vi "OutputSwerve.vi"() -> ()   [LabVIEW 2023]
doc: "This VI runs feedback and feedforward controllers, manages safety interlocks, and sends commands to the swerve drive and azimuth motors. This VI also controls the commanded drive shifter (low gear or high gear) state."
uses:
  d610c66c-71b6-4d3a-a8b1-b399ee96c8a2.vi
  77f8b8d5-fd7b-4b62-a195-6ccd341d14a1.vi
  e7293d0b-e8ab-4975-ac5b-493dfa430016.vi
  4db519e9-bae7-49f3-a1c3-53a7204bbb79.vi
  6abf8b40-ef0a-49e3-8d46-47362e9bd307.vi
  ae5b7493-7bbf-44c5-8d67-5f44d96a3e48.vi
  744fb9e7-64fc-4bc7-b371-cd49665d8c00.vi
  bd7bff45-d105-4c72-b52f-b7d898b15bf8.vi
  GlobalDriverStationData.vi
  GlobalDrivebase.vi
  GRNF_CTREMotor.vi
  GRNF_GenericSolenoid.vi
  TAI_Motor.vi
  TAI_Solenoid.vi
panel:
  in  "Force To High Gear":bool
  in  "Time Below Speed (ms)":u32=150
  in  "Time Above Speed (ms)":u32=150
  in  "Switch to Low Gear (rpm)":dbl=500.0
  in  "Switch to High Gear (rpm)":dbl=4000.0
  in  "Motor Balancing 3":dbl=0.99
  in  "Motor Balancing 2":dbl=1.0
  in  "Motor Balancing 1":dbl=0.9299999999999999
  in  "Motor Balancing 0":dbl=0.97
  in  "Azimuth PID Parameters":T1={"Kp"=0.2, "Ki"=0.0, "Kd"=10.0, "Kf (don't use)"=0.0, "I-Zone"=10.0} {"Kd" min=0.0; "Ki" min=0.0; "Kp" min=0.0}
  in  "Manual Azimuth Goal (deg) [-180,180]":dbl step=5.0
  in  "Manually Override Azimuth Goal":bool
  in  "Best Angle Hysteresis (deg)":dbl=10.0 format="%#_13g"
  out "Azimuth Position":cluster{dbl, "Interlock Output":dbl}(graph)
  out "Azimuth Error (deg)":dbl
  in  "Plotting":T2(ring)
  in  "Force to Low Gear":bool
  in  "Drive Command Override [0,1]":dbl min=0.0 max=1.0 step=0.1
  in  "Manually Override Drive Command":bool
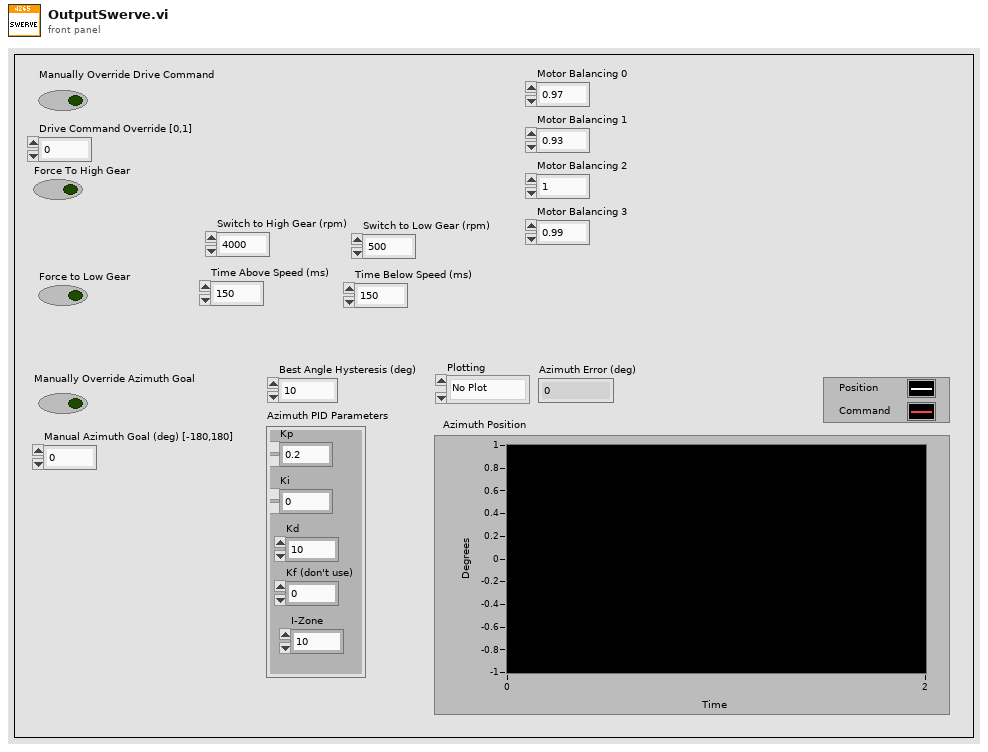
[diagram p1: front panel]
types:
  T1 = cluster{"Kp":dbl, "Ki":dbl, "Kd":dbl, "Kf (don't use)":dbl, "I-Zone":dbl}
  T2 = enum16{"No Plot", "Module 0", "Module 1", "Module 2", "Module 3"}
  T3 = enum16{"Safety", "Travelling", "Positioning", "Holding"}
  T4 = typedef "WPI_MotorControlDeviceRef.ctl" = cluster{"DeviceStatus":errorcluster, "Type":T5, "PWM":cluster{"PWM Channel":T6, "DeadBand":T7}, "CAN":cluster{"Device Number":u8, "SetOutput VI Ref":variant, "GetOutput VI Ref":variant, "Enable VI Ref":variant, "Disable VI Ref":variant, "Data":variant}, "Invert":bool, "DIO PWM":cluster{"PWM \"Enable\" Channel":T6, "DIOChannel":T8, "PWM Rate":dbl}}
  T5 = typedef "WPI_MotorControlType.ctl" = enum16{"PWM", "CAN", "DIO PWM"}
  T6 = typedef "FPGA_DIOPWMChannel.ctl" = enum8{"PWM 0", "PWM 1", "PWM 2", "PWM 3", "PWM 4", "PWM 5", "PWM 6", "PWM 7", "PWM 8", "PWM 9", "PWM MXP 0", "PWM MXP 1", "PWM MXP 2", "PWM MXP 3", "PWM MXP 4", "PWM MXP 5", "PWM MXP 6", "PWM MXP 7", "PWM MXP 8", "PWM MXP 9", "Invalid"}
  T7 = typedef "WPI_PWMDeadband.ctl" = cluster{"Name":string, "maxPositivePwm":i32, "minPositivePwm":i32, "centerPwm":i32, "maxNegativePwm":i32, "minNegativePwm":i32, "angularRange":u16}
  T8 = typedef "FPGA_DIOChannel.ctl" = enum8{"DIO 0", "DIO 1", "DIO 2", "DIO 3", "DIO 4", "DIO 5", "DIO 6", "DIO 7", "DIO 8", "DIO 9", "DIO MXP 0", "DIO MXP 1", "DIO MXP 2", "DIO MXP 3", "DIO MXP 4", "DIO MXP 5", "DIO MXP 6", "DIO MXP 7", "DIO MXP 8", "DIO MXP 9", "DIO MXP 10", "DIO MXP 11", "DIO MXP 12", "DIO MXP 13", "DIO MXP 14", "DIO MXP 15", "SPI Port CS1", "SPI Port CS2", "SPI Port CS3", "SPI Port MISO", "SPI Port MOSI", "Invalid"}
  T9 = enum16{"No Changed Output", "New Normal Output", "New Testing Output"}
  T10 = enum16{"Low Gear", "High Gear", "Transiting", "Unknown", "Force Low Gear"}
  T11 = cluster{"SEN_Azimuth_Position_Unwrapped_3 (deg)":dbl, dbl}
  T12 = typedef "WPI_SolenoidDevRef.ctl" = cluster{"DevStatus":errorcluster, "Pneumatics Control Module":u8, "Forward Solenoid Channel":T13, "Reverse Solenoid Channel":T13}
  T13 = typedef "WPI_SolenoidChannel.ctl" = enum8{"Solenoid 0", "Solenoid 1", "Solenoid 2", "Solenoid 3", "Solenoid 4", "Solenoid 5", "Solenoid 6", "Solenoid 7", "Solenoid 8", "Solenoid 9", "Solenoid 10", "Solenoid 11", "Solenoid 12", "Solenoid 13", "Solenoid 14", "Solenoid 15", "Invalid"}
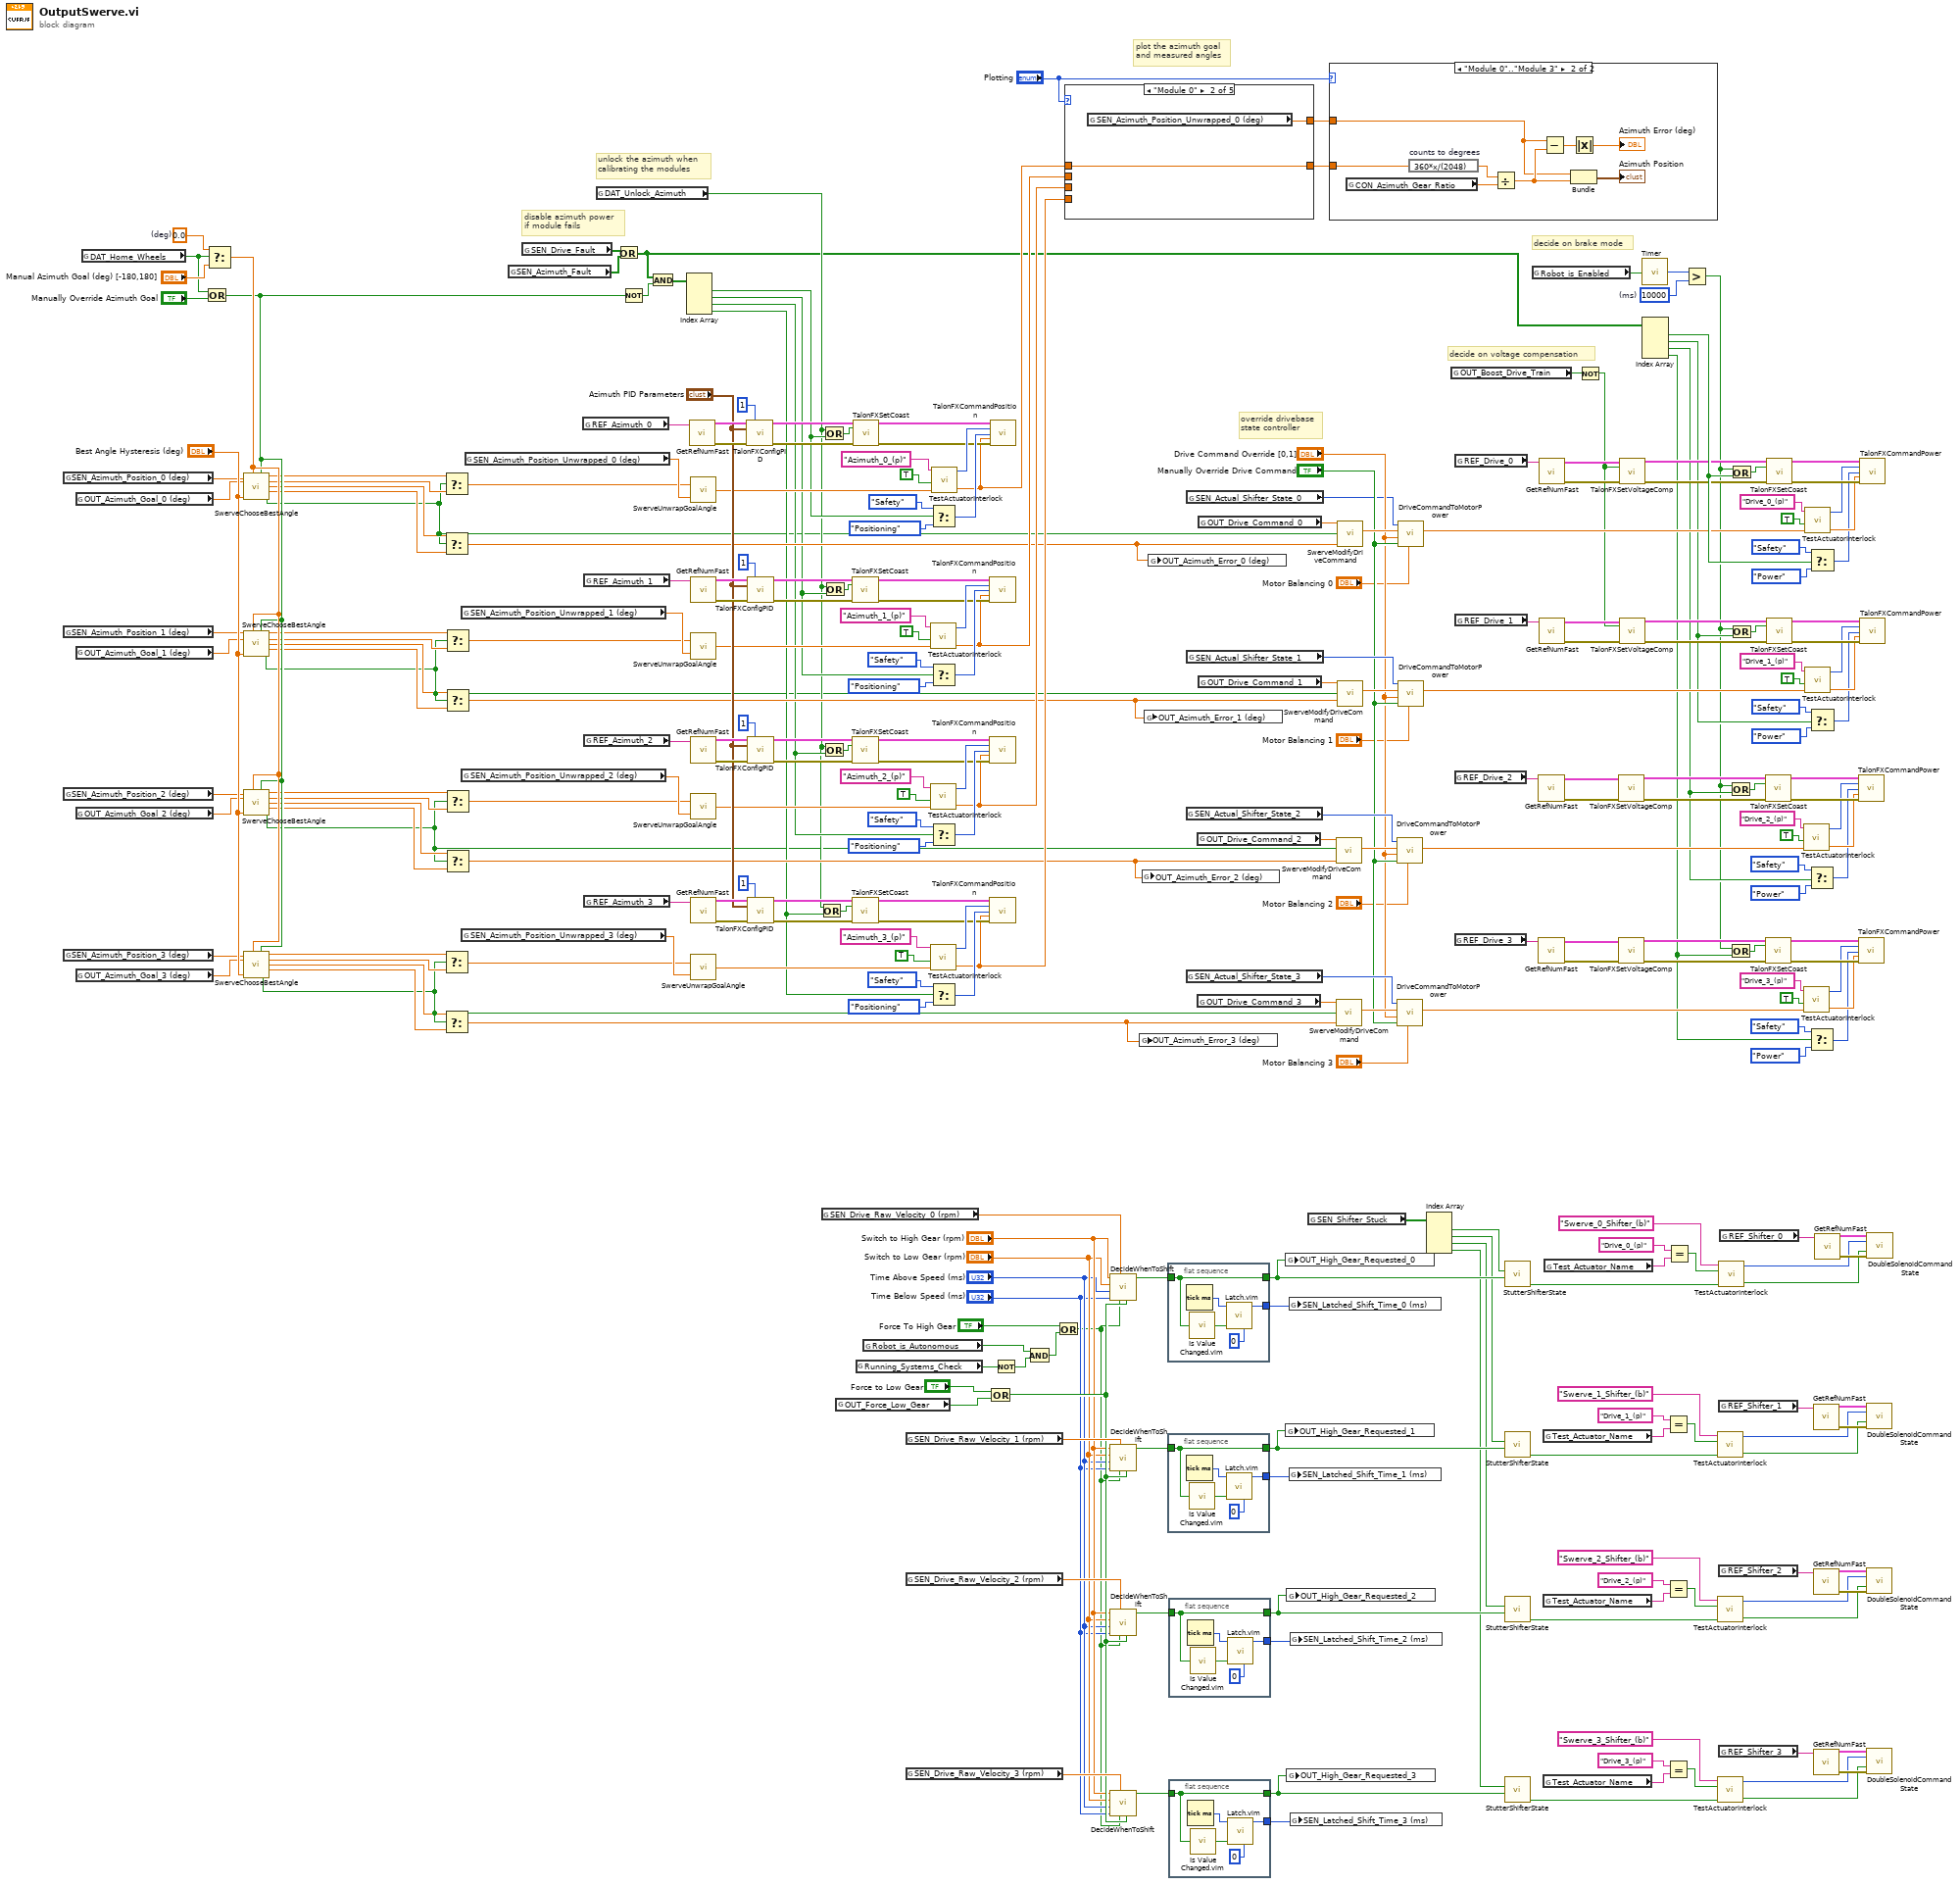
[diagram p0: block diagram]
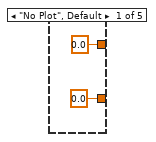
[diagram p3: hidden frame]
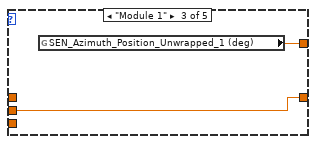
[diagram p4: hidden frame]
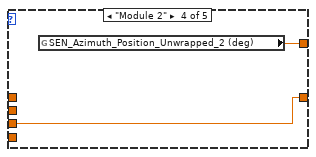
[diagram p5: hidden frame]
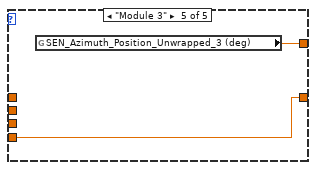
[diagram p6: hidden frame]
diagram:
  w172 = 0.0  # (deg)
  w283 = u32 10000  # (ms)
  # "unlock the azimuth when\ncalibrating the modules"
  # "plot the azimuth goal\nand measured angles"
  # "disable azimuth power\nif module fails"
  # "override drivebase\nstate controller"
  # "decide on brake mode"
  # "decide on voltage compensation"
  n1 = global read "GlobalDrivebase.vi" "SEN_Azimuth_Position_0 (deg)"() -> (w49:dbl)
  n2 = global read "GlobalDrivebase.vi" "SEN_Azimuth_Position_1 (deg)"() -> (w160:dbl)
  n3 = global read "GlobalDrivebase.vi" "SEN_Azimuth_Position_2 (deg)"() -> (w158:dbl)
  n4 = global read "GlobalDrivebase.vi" "SEN_Azimuth_Position_3 (deg)"() -> (w156:dbl)
  n5 = global read "GlobalDrivebase.vi" "OUT_Azimuth_Goal_0 (deg)"() -> (w47:dbl)
  n6 = global read "GlobalDrivebase.vi" "OUT_Azimuth_Goal_1 (deg)"() -> (w164:dbl)
  n7 = global read "GlobalDrivebase.vi" "OUT_Azimuth_Goal_2 (deg)"() -> (w163:dbl)
  n8 = global read "GlobalDrivebase.vi" "OUT_Azimuth_Goal_3 (deg)"() -> (w162:dbl)
  n9 = global read "GlobalDrivebase.vi" "DAT_Home_Wheels"() -> (w96:bool)
  n10 = Or(x=w96, y="Manually Override Azimuth Goal") -> (x .or. y?=w166:bool)
  n11 = Select(t=w172, s=w96, f="Manual Azimuth Goal (deg) [-180,180]") -> (s? t:f=w171:dbl)
  n12 = call "SwerveChooseBestAngle.vi"("Current Angle (deg) [-180,+180]"=w49, "Goal Override Angle (deg) [-180,+180]"=w171, "Goal Override"=w166, "Goal Angle (deg) [-180,+180]"=w47, "Hysteresis (deg)"="Best Angle Hysteresis (deg)") -> ("Flipped Goal Angle (deg) [-180, +180]"=w84:dbl, "Goal Angle (deg) [-180, +180]"=w83:dbl, "Flipped Angular Distance (deg)"=w82:dbl, "Angular Distance (deg)"=w81:dbl, "Flip Drive Motor Direction"=w44:bool)  [unwired: 6 in]
  n13 = call "SwerveChooseBestAngle.vi"("Current Angle (deg) [-180,+180]"=w160, "Goal Override Angle (deg) [-180,+180]"=w171, "Goal Override"=w166, "Goal Angle (deg) [-180,+180]"=w164, "Hysteresis (deg)"="Best Angle Hysteresis (deg)") -> ("Flipped Goal Angle (deg) [-180, +180]"=w80:dbl, "Goal Angle (deg) [-180, +180]"=w79:dbl, "Flipped Angular Distance (deg)"=w77:dbl, "Angular Distance (deg)"=w76:dbl, "Flip Drive Motor Direction"=w45:bool)  [unwired: 6 in]
  n14 = call "SwerveChooseBestAngle.vi"("Current Angle (deg) [-180,+180]"=w158, "Goal Override Angle (deg) [-180,+180]"=w171, "Goal Override"=w166, "Goal Angle (deg) [-180,+180]"=w163, "Hysteresis (deg)"="Best Angle Hysteresis (deg)") -> ("Flipped Goal Angle (deg) [-180, +180]"=w75:dbl, "Goal Angle (deg) [-180, +180]"=w74:dbl, "Flipped Angular Distance (deg)"=w73:dbl, "Angular Distance (deg)"=w72:dbl, "Flip Drive Motor Direction"=w46:bool)  [unwired: 6 in]
  n15 = call "SwerveChooseBestAngle.vi"("Current Angle (deg) [-180,+180]"=w156, "Goal Override Angle (deg) [-180,+180]"=w171, "Goal Override"=w166, "Goal Angle (deg) [-180,+180]"=w162, "Hysteresis (deg)"="Best Angle Hysteresis (deg)") -> ("Flipped Goal Angle (deg) [-180, +180]"=w70:dbl, "Goal Angle (deg) [-180, +180]"=w69:dbl, "Flipped Angular Distance (deg)"=w68:dbl, "Angular Distance (deg)"=w67:dbl, "Flip Drive Motor Direction"=w43:bool)  [unwired: 6 in]
  n16 = Select(t=w84, s=w44, f=w83) -> (s? t:f=w48:dbl)
  n17 = Select(t=w82, s=w44, f=w81) -> (s? t:f=w65:dbl)
  n18 = Select(t=w70, s=w43, f=w69) -> (s? t:f=w66:dbl)
  n19 = Select(t=w68, s=w43, f=w67) -> (s? t:f=w62:dbl)
  n20 = Select(t=w80, s=w45, f=w79) -> (s? t:f=w78:dbl)
  n21 = Select(t=w77, s=w45, f=w76) -> (s? t:f=w64:dbl)
  n22 = Select(t=w75, s=w46, f=w74) -> (s? t:f=w71:dbl)
  n23 = Select(t=w73, s=w46, f=w72) -> (s? t:f=w63:dbl)
  n24 = global read "GlobalDrivebase.vi" "SEN_Azimuth_Position_Unwrapped_1 (deg)"() -> (w159:dbl)
  n25 = global read "GlobalDrivebase.vi" "SEN_Azimuth_Position_Unwrapped_2 (deg)"() -> (w157:dbl)
  n26 = global read "GlobalDrivebase.vi" "SEN_Azimuth_Position_Unwrapped_3 (deg)"() -> (w155:dbl)
  n27 = global read "GlobalDrivebase.vi" "SEN_Azimuth_Position_Unwrapped_0 (deg)"() -> (w161:dbl)
  n28 = global read "GlobalDrivebase.vi" "SEN_Azimuth_Fault"() -> (w51:bool[])
  n29 = global read "GlobalDrivebase.vi" "SEN_Drive_Fault"() -> (w52:bool[])
  n30 = global read "GlobalDrivebase.vi" "REF_Azimuth_0"() -> (w173:string)
  n31 = global read "GlobalDrivebase.vi" "REF_Azimuth_1"() -> (w142:string)
  n32 = global read "GlobalDrivebase.vi" "REF_Azimuth_2"() -> (w129:string)
  n33 = global read "GlobalDrivebase.vi" "REF_Azimuth_3"() -> (w114:string)
  n34 = global read "GlobalDrivebase.vi" "DAT_Unlock_Azimuth"() -> (w53:bool)
  n35 = Or(x=w52, y=w51) -> (x .or. y?=w50:bool[])
  n36 = Not(x=w166) -> (.not. x?=w167:bool)
  n37 = And(x=w50, y=w167) -> (x .and. y?=w168:bool[])
  n38 = Index Array(array=w168) -> (element #1=w60:bool, element #2=w58:bool, element #3=w56:bool, element #4=w54:bool)  [unwired: 4 in]
  n39 = call-poly "GetRefNumFast.vi"("RefNum Name"=w173) -> ("Error"=w145:errorcluster, "Device Reference"=w144:T4)  [unwired: 5 in]
  n40 = call "SwerveUnwrapGoalAngle.vi"("Current Unwrapped Angle (deg) [-Inf,+Inf]"=w161, "Flipped Goal Angle (deg) [-180, +180]"=w48) -> ("Absolute Azimuth Position (tics) [-Inf,+Inf]"=w100:dbl)
  n41 = call-poly "GetRefNumFast.vi"("RefNum Name"=w142) -> ("Error"=w133:errorcluster, "Device Reference"=w132:T4)  [unwired: 5 in]
  n42 = call "SwerveUnwrapGoalAngle.vi"("Current Unwrapped Angle (deg) [-Inf,+Inf]"=w159, "Flipped Goal Angle (deg) [-180, +180]"=w78) -> ("Absolute Azimuth Position (tics) [-Inf,+Inf]"=w99:dbl)
  n43 = call-poly "GetRefNumFast.vi"("RefNum Name"=w129) -> ("Error"=w120:errorcluster, "Device Reference"=w119:T4)  [unwired: 5 in]
  n44 = call "SwerveUnwrapGoalAngle.vi"("Current Unwrapped Angle (deg) [-Inf,+Inf]"=w157, "Flipped Goal Angle (deg) [-180, +180]"=w71) -> ("Absolute Azimuth Position (tics) [-Inf,+Inf]"=w98:dbl)
  n45 = call-poly "GetRefNumFast.vi"("RefNum Name"=w114) -> ("Error"=w105:errorcluster, "Device Reference"=w104:T4)  [unwired: 5 in]
  n46 = call "SwerveUnwrapGoalAngle.vi"("Current Unwrapped Angle (deg) [-Inf,+Inf]"=w155, "Flipped Goal Angle (deg) [-180, +180]"=w66) -> ("Absolute Azimuth Position (tics) [-Inf,+Inf]"=w97:dbl)
  n47 = call "TalonFXConfigPID.vi"("Device Reference (in)"=w144, "PID Slot"=1 ("slotIdx"), "PID Parameters"="Azimuth PID Parameters", "Error (in)"=w145) -> ("Device Reference (out)"=w147:T4, "Error (out)"=w146:errorcluster)  [unwired: 10 in]
  n48 = call "TalonFXConfigPID.vi"("Device Reference (in)"=w132, "PID Slot"=1 ("slotIdx"), "PID Parameters"="Azimuth PID Parameters", "Error (in)"=w133) -> ("Device Reference (out)"=w135:T4, "Error (out)"=w134:errorcluster)  [unwired: 10 in]
  n49 = call "TalonFXConfigPID.vi"("Device Reference (in)"=w119, "PID Slot"=1 ("slotIdx"), "PID Parameters"="Azimuth PID Parameters", "Error (in)"=w120) -> ("Device Reference (out)"=w122:T4, "Error (out)"=w121:errorcluster)  [unwired: 10 in]
  n50 = call "TalonFXConfigPID.vi"("Device Reference (in)"=w104, "PID Slot"=1 ("slotIdx"), "PID Parameters"="Azimuth PID Parameters", "Error (in)"=w105) -> ("Device Reference (out)"=w107:T4, "Error (out)"=w106:errorcluster)  [unwired: 10 in]
  n51 = Or(x=w53, y=w54) -> (x .or. y?=w55:bool)
  n52 = Or(x=w53, y=w60) -> (x .or. y?=w61:bool)
  n53 = Or(x=w53, y=w56) -> (x .or. y?=w57:bool)
  n54 = global read "GlobalDrivebase.vi" "SEN_Drive_Raw_Velocity_0 (rpm)"() -> (w35:dbl)
  n55 = Or(x=w53, y=w58) -> (x .or. y?=w59:bool)
  n56 = global read "GlobalDrivebase.vi" "OUT_Force_Low_Gear"() -> (w288:bool)
  n57 = call "TalonFXSetCoast.vi"("Device Reference (in)"=w135, "Set Coast Mode"=w59, "Error (in)"=w134) -> ("Device Reference (out)"=w92:T4, "Error (out)"=w136:errorcluster)  [unwired: 11 in]
  n58 = call "TalonFXSetCoast.vi"("Device Reference (in)"=w122, "Set Coast Mode"=w57, "Error (in)"=w121) -> ("Device Reference (out)"=w91:T4, "Error (out)"=w123:errorcluster)  [unwired: 11 in]
  n59 = call "TalonFXSetCoast.vi"("Device Reference (in)"=w107, "Set Coast Mode"=w55, "Error (in)"=w106) -> ("Device Reference (out)"=w90:T4, "Error (out)"=w108:errorcluster)  [unwired: 11 in]
  n60 = call "TalonFXSetCoast.vi"("Device Reference (in)"=w147, "Set Coast Mode"=w61, "Error (in)"=w146) -> ("Device Reference (out)"=w143:T4, "Error (out)"=w149:errorcluster)  [unwired: 11 in]
  n61 = global read "GlobalDriverStationData.vi" "Running_Systems_Check"() -> (w37:bool)
  n62 = global read "GlobalDriverStationData.vi" "Robot_is_Autonomous"() -> (w38:bool)
  n63 = global read "GlobalDrivebase.vi" "SEN_Drive_Raw_Velocity_1 (rpm)"() -> (w34:dbl)
  n64 = global read "GlobalDrivebase.vi" "SEN_Drive_Raw_Velocity_2 (rpm)"() -> (w33:dbl)
  n65 = global read "GlobalDrivebase.vi" "SEN_Drive_Raw_Velocity_3 (rpm)"() -> (w32:dbl)
  n66 = call-poly "TestActuatorInterlock.vi"("Normal Output"=w99, "Aux Trigger"=TRUE, "Actuator Name"="Azimuth_1_(p)" ("Actuator_Name")) -> ("Interlocked Output"=w130:dbl, "Testing Mode"=w140:T9)  [unwired: 2 in]
  n67 = Select(t=T3."Safety" ("Control Mode"), s=w58, f=T3."Positioning") -> (s? t:f=w137:T3)
  n68 = call-poly "TestActuatorInterlock.vi"("Normal Output"=w98, "Aux Trigger"=TRUE, "Actuator Name"="Azimuth_2_(p)" ("Actuator_Name")) -> ("Interlocked Output"=w94:dbl, "Testing Mode"=w127:T9)  [unwired: 2 in]
  n69 = Select(t=T3."Safety" ("Control Mode"), s=w56, f=T3."Positioning") -> (s? t:f=w124:T3)
  n70 = call-poly "TestActuatorInterlock.vi"("Normal Output"=w97, "Aux Trigger"=TRUE, "Actuator Name"="Azimuth_3_(p)" ("Actuator_Name")) -> ("Interlocked Output"=w93:dbl, "Testing Mode"=w112:T9)  [unwired: 2 in]
  n71 = Select(t=T3."Safety" ("Control Mode"), s=w54, f=T3."Positioning") -> (s? t:f=w109:T3)
  n72 = call-poly "TestActuatorInterlock.vi"("Normal Output"=w100, "Aux Trigger"=TRUE, "Actuator Name"="Azimuth_0_(p)" ("Actuator_Name")) -> ("Interlocked Output"=w87:dbl, "Testing Mode"=w153:T9)  [unwired: 2 in]
  n73 = Select(t=T3."Safety" ("Control Mode"), s=w60, f=T3."Positioning") -> (s? t:f=w150:T3)
  n74 = call "TalonFXCommandPosition.vi"("Device Reference (in)"=w92, "Output Mode"=w140, "Control Mode"=w137, "Position (counts) or Testing Power"=w130, "Error (in)"=w136) -> ()  [unwired: 11 in]
  n75 = call "TalonFXCommandPosition.vi"("Device Reference (in)"=w91, "Output Mode"=w127, "Control Mode"=w124, "Position (counts) or Testing Power"=w94, "Error (in)"=w123) -> ()  [unwired: 11 in]
  n76 = call "TalonFXCommandPosition.vi"("Device Reference (in)"=w90, "Output Mode"=w112, "Control Mode"=w109, "Position (counts) or Testing Power"=w93, "Error (in)"=w108) -> ()  [unwired: 11 in]
  n77 = call "TalonFXCommandPosition.vi"("Device Reference (in)"=w143, "Output Mode"=w153, "Control Mode"=w150, "Position (counts) or Testing Power"=w87, "Error (in)"=w149) -> ()  [unwired: 11 in]
  n78 = Compound Arithmetic op=OR("Force to Low Gear", w288) -> (w31:bool)
  n79 = Not(x=w37) -> (.not. x?=w36:bool)
  n80 = Compound Arithmetic op=AND(w38, w36) -> (w17:bool)
  n81 = Or(x="Force To High Gear", y=w17) -> (x .or. y?=w15:bool)
  n82 = case shown="\"Module 0\"" "Plotting" {
    tunnel: w87 -> [_ w299 _ _ _]
    tunnel: [0.0 ("Interlock Output") w299 w300 w303 w305] -> w169
    tunnel: w130 -> [_ _ w300 _ _]
    tunnel: w94 -> [_ _ _ w303 _]
    tunnel: w93 -> [_ _ _ _ w305]
    tunnel: [0.0 ("SEN_Azimuth_Position_Unwrapped_3 (deg)") w298 w301 w302 w304] -> w89
    frame "No Plot", Default {
    }
    frame "Module 0" {
      n83 = global read "GlobalDrivebase.vi" "SEN_Azimuth_Position_Unwrapped_0 (deg)"() -> (w298:dbl)
    }
    frame "Module 1" {
      n84 = global read "GlobalDrivebase.vi" "SEN_Azimuth_Position_Unwrapped_1 (deg)"() -> (w301:dbl)
    }
    frame "Module 2" {
      n85 = global read "GlobalDrivebase.vi" "SEN_Azimuth_Position_Unwrapped_2 (deg)"() -> (w302:dbl)
    }
    frame "Module 3" {
      n86 = global read "GlobalDrivebase.vi" "SEN_Azimuth_Position_Unwrapped_3 (deg)"() -> (w304:dbl)
    }
  }
  n87 = call "DecideWhenToShift.vi"("Force to Low Gear"=w31, "Force To High Gear"=w15, "Drive Motor Speed (rpm)"=w35, "Time Below Speed (ms)"="Time Below Speed (ms)", "Time Above Speed (ms)"="Time Above Speed (ms)", "Switch to Low Gear (rpm)"="Switch to Low Gear (rpm)", "Switch to High Gear (rpm)"="Switch to High Gear (rpm)") -> ("Requested Shifter State"=w294:bool)  [unwired: 4 in]
  n88 = call "DecideWhenToShift.vi"("Force to Low Gear"=w31, "Force To High Gear"=w15, "Drive Motor Speed (rpm)"=w34, "Time Below Speed (ms)"="Time Below Speed (ms)", "Time Above Speed (ms)"="Time Above Speed (ms)", "Switch to Low Gear (rpm)"="Switch to Low Gear (rpm)", "Switch to High Gear (rpm)"="Switch to High Gear (rpm)") -> ("Requested Shifter State"=w178:bool)  [unwired: 4 in]
  n89 = call "DecideWhenToShift.vi"("Force to Low Gear"=w31, "Force To High Gear"=w15, "Drive Motor Speed (rpm)"=w33, "Time Below Speed (ms)"="Time Below Speed (ms)", "Time Above Speed (ms)"="Time Above Speed (ms)", "Switch to Low Gear (rpm)"="Switch to Low Gear (rpm)", "Switch to High Gear (rpm)"="Switch to High Gear (rpm)") -> ("Requested Shifter State"=w176:bool)  [unwired: 4 in]
  n90 = call "DecideWhenToShift.vi"("Force to Low Gear"=w31, "Force To High Gear"=w15, "Drive Motor Speed (rpm)"=w32, "Time Below Speed (ms)"="Time Below Speed (ms)", "Time Above Speed (ms)"="Time Above Speed (ms)", "Switch to Low Gear (rpm)"="Switch to Low Gear (rpm)", "Switch to High Gear (rpm)"="Switch to High Gear (rpm)") -> ("Requested Shifter State"=w174:bool)  [unwired: 4 in]
  n91 = global write "GlobalDrivebase.vi" "OUT_Azimuth_Error_3 (deg)"(w62) -> ()
  n92 = global write "GlobalDrivebase.vi" "OUT_Azimuth_Error_2 (deg)"(w63) -> ()
  n93 = global write "GlobalDrivebase.vi" "OUT_Azimuth_Error_1 (deg)"(w64) -> ()
  n94 = global write "GlobalDrivebase.vi" "OUT_Azimuth_Error_0 (deg)"(w65) -> ()
  n95 = flat-sequence {
    tunnel: w294 -> [w308]
    tunnel: [w308] -> w9
    tunnel: [w306] -> w180
    frame #0 {
      n96 = Tick Count (ms)() -> (millisecond timer value=w310:u32)
      n97 = call "Is Value Changed.vim"("value"=w308) -> ("changed or first call?"=w307:bool)
      n98 = call "Latch.vim"("Default Value"=u32 0 ("millisecond timer value"), "Latch Signal"=w307, "Latch Value"=w310) -> ("Latched"=w306:u32)  [unwired: 8 in]
    }
  }
  n99 = flat-sequence {
    tunnel: w178 -> [w313]
    tunnel: [w313] -> w10
    tunnel: [w311] -> w179
    frame #0 {
      n100 = Tick Count (ms)() -> (millisecond timer value=w315:u32)
      n101 = call "Is Value Changed.vim"("value"=w313) -> ("changed or first call?"=w312:bool)
      n102 = call "Latch.vim"("Default Value"=u32 0 ("millisecond timer value"), "Latch Signal"=w312, "Latch Value"=w315) -> ("Latched"=w311:u32)  [unwired: 8 in]
    }
  }
  n103 = flat-sequence {
    tunnel: w176 -> [w318]
    tunnel: [w318] -> w8
    tunnel: [w316] -> w177
    frame #0 {
      n104 = Tick Count (ms)() -> (millisecond timer value=w320:u32)
      n105 = call "Is Value Changed.vim"("value"=w318) -> ("changed or first call?"=w317:bool)
      n106 = call "Latch.vim"("Default Value"=u32 0 ("millisecond timer value"), "Latch Signal"=w317, "Latch Value"=w320) -> ("Latched"=w316:u32)  [unwired: 8 in]
    }
  }
  n107 = flat-sequence {
    tunnel: w174 -> [w323]
    tunnel: [w323] -> w7
    tunnel: [w321] -> w175
    frame #0 {
      n108 = Tick Count (ms)() -> (millisecond timer value=w325:u32)
      n109 = call "Is Value Changed.vim"("value"=w323) -> ("changed or first call?"=w322:bool)
      n110 = call "Latch.vim"("Default Value"=u32 0 ("millisecond timer value"), "Latch Signal"=w322, "Latch Value"=w325) -> ("Latched"=w321:u32)  [unwired: 8 in]
    }
  }
  n111 = global read "GlobalDrivebase.vi" "SEN_Actual_Shifter_State_2"() -> (w248:T10)
  n112 = global read "GlobalDrivebase.vi" "SEN_Actual_Shifter_State_3"() -> (w231:T10)
  n113 = global read "GlobalDrivebase.vi" "SEN_Actual_Shifter_State_0"() -> (w1:T10)
  n114 = global read "GlobalDrivebase.vi" "SEN_Actual_Shifter_State_1"() -> (w266:T10)
  n115 = global read "GlobalDrivebase.vi" "OUT_Drive_Command_2"() -> (w249:dbl)
  n116 = global read "GlobalDrivebase.vi" "OUT_Drive_Command_3"() -> (w232:dbl)
  n117 = global read "GlobalDrivebase.vi" "OUT_Drive_Command_0"() -> (w289:dbl)
  n118 = global read "GlobalDrivebase.vi" "OUT_Drive_Command_1"() -> (w267:dbl)
  n119 = global write "GlobalDrivebase.vi" "OUT_High_Gear_Requested_0"(w9) -> ()
  n120 = global write "GlobalDrivebase.vi" "OUT_High_Gear_Requested_1"(w10) -> ()
  n121 = global write "GlobalDrivebase.vi" "OUT_High_Gear_Requested_2"(w8) -> ()
  n122 = global write "GlobalDrivebase.vi" "OUT_High_Gear_Requested_3"(w7) -> ()
  n123 = global write "GlobalDrivebase.vi" "SEN_Latched_Shift_Time_0 (ms)"(w180) -> ()
  n124 = global write "GlobalDrivebase.vi" "SEN_Latched_Shift_Time_1 (ms)"(w179) -> ()
  n125 = global write "GlobalDrivebase.vi" "SEN_Latched_Shift_Time_2 (ms)"(w177) -> ()
  n126 = global write "GlobalDrivebase.vi" "SEN_Latched_Shift_Time_3 (ms)"(w175) -> ()
  n127 = global read "GlobalDrivebase.vi" "SEN_Shifter_Stuck"() -> (w6:bool[])
  n128 = case shown="\"Module 0\"..\"Module 3\"" "Plotting" {
    tunnel: w169 -> [_ w332]
    tunnel: w89 -> [_ w326]
    frame "No Plot", Default {
    }
    frame "Module 0".."Module 3" {
      n129 = global read "GlobalDrivebase.vi" "CON_Azimuth_Gear_Ratio"() -> (w327:dbl)
      n130 = expression code="360*x/(2048)" "counts to degrees"(w332) -> (w329:dbl)
      n131 = Divide(x=w329, y=w327) -> (x/y=w328:dbl)
      n132 = Subtract(x=w326, y=w328) -> (x-y=w331:dbl)
      n133 = Bundle("SEN_Azimuth_Position_Unwrapped_3 (deg)"=w326, w328) -> (→"Azimuth Position":T11)  [unwired: 1 in]
      n134 = Absolute Value(x=w331) -> (abs(x)=→"Azimuth Error (deg)":dbl)
    }
  }
  n135 = call "SwerveModifyDriveCommand.vi"("Raw Drive Command (ul)"=w249, "Flip Drive Command"=w46, "Azimuth Error (deg)"=w63) -> ("Modified Drive Command (ul)"=w233:dbl)  [unwired: 3 in]
  n136 = call "SwerveModifyDriveCommand.vi"("Raw Drive Command (ul)"=w232, "Flip Drive Command"=w43, "Azimuth Error (deg)"=w62) -> ("Modified Drive Command (ul)"=w216:dbl)  [unwired: 3 in]
  n137 = call "SwerveModifyDriveCommand.vi"("Raw Drive Command (ul)"=w289, "Flip Drive Command"=w44, "Azimuth Error (deg)"=w65) -> ("Modified Drive Command (ul)"=w268:dbl)  [unwired: 3 in]
  n138 = call "SwerveModifyDriveCommand.vi"("Raw Drive Command (ul)"=w267, "Flip Drive Command"=w45, "Azimuth Error (deg)"=w64) -> ("Modified Drive Command (ul)"=w251:dbl)  [unwired: 3 in]
  n139 = call "DriveCommandToMotorPower.vi"("Motor Balancing"="Motor Balancing 2", "Drive Command Override"="Manually Override Drive Command", "Drive Command Override (ul) [-1,1]"="Drive Command Override [0,1]", "Drive Command (ul) [-1,1]"=w233, "Actual Shifter State"=w248) -> ("Motor Power (ul) [-1,1]"=w234:dbl)  [unwired: 6 in]
  n140 = call "DriveCommandToMotorPower.vi"("Motor Balancing"="Motor Balancing 3", "Drive Command Override"="Manually Override Drive Command", "Drive Command Override (ul) [-1,1]"="Drive Command Override [0,1]", "Drive Command (ul) [-1,1]"=w216, "Actual Shifter State"=w231) -> ("Motor Power (ul) [-1,1]"=w217:dbl)  [unwired: 6 in]
  n141 = call "DriveCommandToMotorPower.vi"("Motor Balancing"="Motor Balancing 0", "Drive Command Override"="Manually Override Drive Command", "Drive Command Override (ul) [-1,1]"="Drive Command Override [0,1]", "Drive Command (ul) [-1,1]"=w268, "Actual Shifter State"=w1) -> ("Motor Power (ul) [-1,1]"=w269:dbl)  [unwired: 6 in]
  n142 = call "DriveCommandToMotorPower.vi"("Motor Balancing"="Motor Balancing 1", "Drive Command Override"="Manually Override Drive Command", "Drive Command Override (ul) [-1,1]"="Drive Command Override [0,1]", "Drive Command (ul) [-1,1]"=w251, "Actual Shifter State"=w266) -> ("Motor Power (ul) [-1,1]"=w252:dbl)  [unwired: 6 in]
  n143 = Index Array(array=w6) -> (element #1=w2:bool, element #2=w4:bool, element #3=w3:bool, element #4=w5:bool)  [unwired: 4 in]
  n144 = global read "GlobalDrivebase.vi" "OUT_Boost_Drive_Train"() -> (w270:bool)
  n145 = global read "GlobalDrivebase.vi" "REF_Drive_2"() -> (w246:string)
  n146 = global read "GlobalDrivebase.vi" "REF_Drive_3"() -> (w229:string)
  n147 = global read "GlobalDrivebase.vi" "REF_Drive_0"() -> (w286:string)
  n148 = global read "GlobalDrivebase.vi" "REF_Drive_1"() -> (w264:string)
  n149 = call "StutterShifterState.vi"("Requested Shifter State"=w9, "Request Stutter"=w2) -> ("Stuttered Shifter State"=w11:bool)  [unwired: 9 in]
  n150 = call "StutterShifterState.vi"("Requested Shifter State"=w10, "Request Stutter"=w4) -> ("Stuttered Shifter State"=w12:bool)  [unwired: 9 in]
  n151 = call "StutterShifterState.vi"("Requested Shifter State"=w8, "Request Stutter"=w3) -> ("Stuttered Shifter State"=w13:bool)  [unwired: 9 in]
  n152 = call "StutterShifterState.vi"("Requested Shifter State"=w7, "Request Stutter"=w5) -> ("Stuttered Shifter State"=w14:bool)  [unwired: 9 in]
  n153 = global read "GlobalDriverStationData.vi" "Robot_is_Enabled"() -> (w282:bool)
  n154 = call-poly "GetRefNumFast.vi"("RefNum Name"=w246) -> ("Error"=w237:errorcluster, "Device Reference"=w238:T4)  [unwired: 5 in]
  n155 = call-poly "GetRefNumFast.vi"("RefNum Name"=w229) -> ("Error"=w220:errorcluster, "Device Reference"=w221:T4)  [unwired: 5 in]
  n156 = call-poly "GetRefNumFast.vi"("RefNum Name"=w286) -> ("Error"=w273:errorcluster, "Device Reference"=w274:T4)  [unwired: 5 in]
  n157 = call-poly "GetRefNumFast.vi"("RefNum Name"=w264) -> ("Error"=w255:errorcluster, "Device Reference"=w256:T4)  [unwired: 5 in]
  n158 = global read "GlobalDriverStationData.vi" "Test_Actuator_Name"() -> (w205:string)
  n159 = global read "GlobalDriverStationData.vi" "Test_Actuator_Name"() -> (w196:string)
  n160 = global read "GlobalDriverStationData.vi" "Test_Actuator_Name"() -> (w187:string)
  n161 = global read "GlobalDriverStationData.vi" "Test_Actuator_Name"() -> (w291:string)
  n162 = Not(x=w270) -> (.not. x?=w250:bool)
  n163 = call "TalonFXSetVoltageComp.vi"("Device Reference (in)"=w238, "Error (in)"=w237) -> ("Device Reference (out)"=w236:T4, "Error (out)"=w235:errorcluster)  [unwired: 12 in]
  n164 = call "TalonFXSetVoltageComp.vi"("Device Reference (in)"=w221, "Error (in)"=w220) -> ("Device Reference (out)"=w219:T4, "Error (out)"=w218:errorcluster)  [unwired: 12 in]
  n165 = call "TalonFXSetVoltageComp.vi"("Device Reference (in)"=w274, "Set Voltage Compensation Mode"=w250, "Error (in)"=w273) -> ("Device Reference (out)"=w272:T4, "Error (out)"=w271:errorcluster)  [unwired: 11 in]
  n166 = call "TalonFXSetVoltageComp.vi"("Device Reference (in)"=w256, "Set Voltage Compensation Mode"=w250, "Error (in)"=w255) -> ("Device Reference (out)"=w254:T4, "Error (out)"=w253:errorcluster)  [unwired: 11 in]
  n167 = call "Timer.vi"("Reset Timer"=w282) -> ("Time (ms)"=w284:u32)
  n168 = Index Array(array=w50) -> (element #1=w275:bool, element #2=w213:bool, element #3=w86:bool, element #4=w85:bool)  [unwired: 4 in]
  n169 = Equal?(x="Drive_1_(p)" ("Actuator_Name"), y=w205) -> (x = y?=w204:bool)
  n170 = Equal?(x="Drive_2_(p)" ("Actuator_Name"), y=w196) -> (x = y?=w195:bool)
  n171 = Equal?(x="Drive_3_(p)" ("Actuator_Name"), y=w187) -> (x = y?=w186:bool)
  n172 = Equal?(x="Drive_0_(p)" ("Actuator_Name"), y=w291) -> (x = y?=w290:bool)
  n173 = Greater?(x=w284, y=w283) -> (0:w18:bool)
  n174 = call-poly "TestActuatorInterlock.vi"("Normal Output"=w12, "Override Actuator Bypass"=w204, "Actuator Name"="Swerve_1_Shifter_(b)" ("Actuator_Name")) -> ("Interlocked Output"=w199:bool, "Output Mode"=w200:T9)  [unwired: 2 in]
  n175 = call-poly "TestActuatorInterlock.vi"("Normal Output"=w13, "Override Actuator Bypass"=w195, "Actuator Name"="Swerve_2_Shifter_(b)" ("Actuator_Name")) -> ("Interlocked Output"=w190:bool, "Output Mode"=w191:T9)  [unwired: 2 in]
  n176 = call-poly "TestActuatorInterlock.vi"("Normal Output"=w14, "Override Actuator Bypass"=w186, "Actuator Name"="Swerve_3_Shifter_(b)" ("Actuator_Name")) -> ("Interlocked Output"=w181:bool, "Output Mode"=w182:T9)  [unwired: 2 in]
  n177 = call-poly "TestActuatorInterlock.vi"("Normal Output"=w11, "Override Actuator Bypass"=w290, "Actuator Name"="Swerve_0_Shifter_(b)" ("Actuator_Name")) -> ("Interlocked Output"=w208:bool, "Output Mode"=w209:T9)  [unwired: 2 in]
  n178 = global read "GlobalDrivebase.vi" "REF_Shifter_1"() -> (w203:string)
  n179 = global read "GlobalDrivebase.vi" "REF_Shifter_2"() -> (w194:string)
  n180 = global read "GlobalDrivebase.vi" "REF_Shifter_3"() -> (w185:string)
  n181 = global read "GlobalDrivebase.vi" "REF_Shifter_0"() -> (w212:string)
  n182 = Or(x=w18, y=w86) -> (x .or. y?=w245:bool)
  n183 = Or(x=w18, y=w85) -> (x .or. y?=w228:bool)
  n184 = Or(x=w18, y=w275) -> (x .or. y?=w285:bool)
  n185 = Or(x=w18, y=w213) -> (x .or. y?=w263:bool)
  n186 = call "TalonFXSetCoast.vi"("Device Reference (in)"=w236, "Set Coast Mode"=w245, "Error (in)"=w235) -> ("Device Reference (out)"=w243:T4, "Error (out)"=w242:errorcluster)  [unwired: 11 in]
  n187 = call "TalonFXSetCoast.vi"("Device Reference (in)"=w219, "Set Coast Mode"=w228, "Error (in)"=w218) -> ("Device Reference (out)"=w226:T4, "Error (out)"=w225:errorcluster)  [unwired: 11 in]
  n188 = call "TalonFXSetCoast.vi"("Device Reference (in)"=w272, "Set Coast Mode"=w285, "Error (in)"=w271) -> ("Device Reference (out)"=w280:T4, "Error (out)"=w279:errorcluster)  [unwired: 11 in]
  n189 = call "TalonFXSetCoast.vi"("Device Reference (in)"=w254, "Set Coast Mode"=w263, "Error (in)"=w253) -> ("Device Reference (out)"=w261:T4, "Error (out)"=w260:errorcluster)  [unwired: 11 in]
  n190 = call-poly "TestActuatorInterlock.vi"("Normal Output"=w234, "Aux Trigger"=TRUE, "Actuator Name"="Drive_2_(p)" ("Actuator_Name")) -> ("Interlocked Output"=w241:dbl, "Testing Mode"=w240:T9)  [unwired: 2 in]
  n191 = call-poly "TestActuatorInterlock.vi"("Normal Output"=w217, "Aux Trigger"=TRUE, "Actuator Name"="Drive_3_(p)" ("Actuator_Name")) -> ("Interlocked Output"=w224:dbl, "Testing Mode"=w223:T9)  [unwired: 2 in]
  n192 = call-poly "TestActuatorInterlock.vi"("Normal Output"=w269, "Aux Trigger"=TRUE, "Actuator Name"="Drive_0_(p)" ("Actuator_Name")) -> ("Interlocked Output"=w278:dbl, "Testing Mode"=w277:T9)  [unwired: 2 in]
  n193 = call-poly "TestActuatorInterlock.vi"("Normal Output"=w252, "Aux Trigger"=TRUE, "Actuator Name"="Drive_1_(p)" ("Actuator_Name")) -> ("Interlocked Output"=w259:dbl, "Testing Mode"=w258:T9)  [unwired: 2 in]
  n194 = Select(t=enum16{"Safety", "Power"}."Safety" ("Control Mode"), s=w86, f=enum16{"Safety", "Power"}."Power") -> (s? t:f=w23:enum16{"Safety", "Power"})
  n195 = Select(t=enum16{"Safety", "Power"}."Safety" ("Control Mode"), s=w85, f=enum16{"Safety", "Power"}."Power") -> (s? t:f=w25:enum16{"Safety", "Power"})
  n196 = Select(t=enum16{"Safety", "Power"}."Safety" ("Control Mode"), s=w275, f=enum16{"Safety", "Power"}."Power") -> (s? t:f=w19:enum16{"Safety", "Power"})
  n197 = Select(t=enum16{"Safety", "Power"}."Safety" ("Control Mode"), s=w213, f=enum16{"Safety", "Power"}."Power") -> (s? t:f=w21:enum16{"Safety", "Power"})
  n198 = call-poly "GetRefNumFast.vi"("RefNum Name"=w203) -> ("Error"=w201:errorcluster, "Device Reference"=w202:T12)  [unwired: 5 in]
  n199 = call-poly "GetRefNumFast.vi"("RefNum Name"=w194) -> ("Error"=w192:errorcluster, "Device Reference"=w193:T12)  [unwired: 5 in]
  n200 = call-poly "GetRefNumFast.vi"("RefNum Name"=w185) -> ("Error"=w183:errorcluster, "Device Reference"=w184:T12)  [unwired: 5 in]
  n201 = call-poly "GetRefNumFast.vi"("RefNum Name"=w212) -> ("Error"=w210:errorcluster, "Device Reference"=w211:T12)  [unwired: 5 in]
  n202 = call "TalonFXCommandPower.vi"("Device Reference (in)"=w243, "Output Mode"=w240, "Control Mode"=w23, "Power or Testing Power"=w241, "Error (in)"=w242) -> ()  [unwired: 11 in]
  n203 = call "TalonFXCommandPower.vi"("Device Reference (in)"=w226, "Output Mode"=w223, "Control Mode"=w25, "Power or Testing Power"=w224, "Error (in)"=w225) -> ()  [unwired: 11 in]
  n204 = call "TalonFXCommandPower.vi"("Device Reference (in)"=w280, "Output Mode"=w277, "Control Mode"=w19, "Power or Testing Power"=w278, "Error (in)"=w279) -> ()  [unwired: 11 in]
  n205 = call "TalonFXCommandPower.vi"("Device Reference (in)"=w261, "Output Mode"=w258, "Control Mode"=w21, "Power or Testing Power"=w259, "Error (in)"=w260) -> ()  [unwired: 11 in]
  n206 = call "DoubleSolenoidCommandState.vi"("Device Reference (in)"=w202, "Output Mode"=w200, "State [True, False]"=w199, "Error (in)"=w201) -> ()  [unwired: 12 in]
  n207 = call "DoubleSolenoidCommandState.vi"("Device Reference (in)"=w193, "Output Mode"=w191, "State [True, False]"=w190, "Error (in)"=w192) -> ()  [unwired: 12 in]
  n208 = call "DoubleSolenoidCommandState.vi"("Device Reference (in)"=w184, "Output Mode"=w182, "State [True, False]"=w181, "Error (in)"=w183) -> ()  [unwired: 12 in]
  n209 = call "DoubleSolenoidCommandState.vi"("Device Reference (in)"=w211, "Output Mode"=w209, "State [True, False]"=w208, "Error (in)"=w210) -> ()  [unwired: 12 in]
